vi "Write Sub Nodes.vi"(8 "error in (no error)":errorcluster, 10 "Sub Nodes":refnum<class "Tree Data.lvclass">[](array[class]), 11 "Composite Tree Data in":refnum<class "Composite Tree Data.lvclass">) -> (0 "error out":errorcluster, 3 "Composite Tree Data out":refnum<class "Composite Tree Data.lvclass">)   [LabVIEW 2024, in "Composite Tree Data.lvclass"]
uses:
  Composite Tree Data.lvclass
  Tree Data/Tree Data.lvclass
  Composite Tree Data.lvclass/Composite Tree Data.ctl
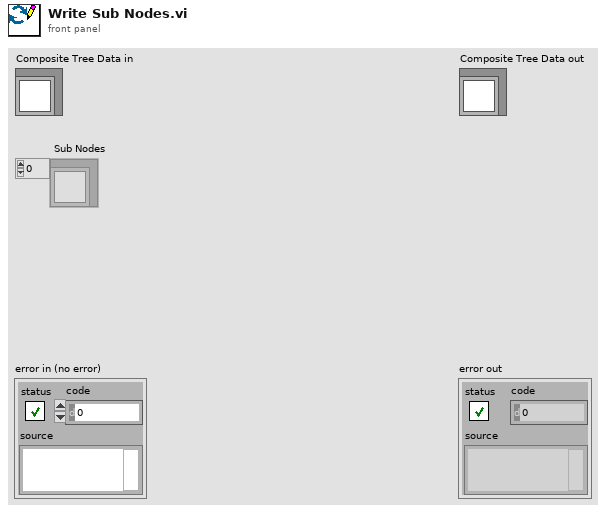
[diagram p1: front panel]
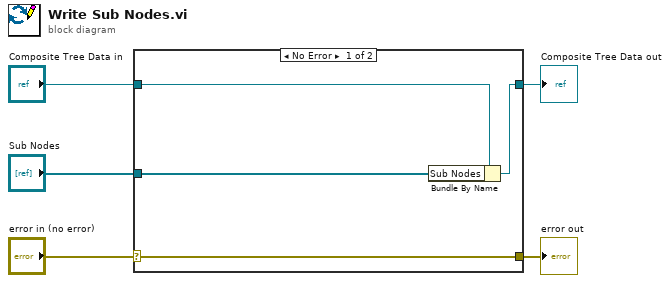
[diagram p0: block diagram]
diagram:
  n1 = case shown="No Error" "error in (no error)" {
    selector: "error in (no error)" -> [w9 w10]
    tunnel: [w9 w10] -> w4
    tunnel: [w7 w11] -> w2
    tunnel: "Composite Tree Data in" -> [w8 w11]
    tunnel: "Sub Nodes" -> [w6 _]
    frame No Error {
      n2 = Bundle By Name(cluster=w8, "Sub Nodes"=w6) -> (w7:refnum<class "Composite Tree Data.lvclass">)
    }
    frame Error {
    }
  }
  "error out" <- w4
  "Composite Tree Data out" <- w2
